vi "Write Message Queue.vi"(10 "Message Queue":refnum<class "JQMH_Message Queue.lvclass">, 11 "JQMHModule in":refnum<class "JQMHModule.lvclass">) -> (3 "JQMHModule out":refnum<class "JQMHModule.lvclass">)   [LabVIEW 2024, in "JQMHModule.lvclass"]
uses:
  JQMHModule.lvclass
  JQMHModule.lvclass/JQMHModule.ctl
  Message Queue_class/JQMH_Message Queue.lvclass
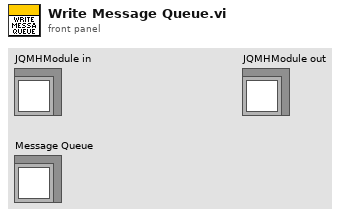
[diagram p1: front panel]
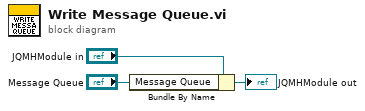
[diagram p0: block diagram]
diagram:
  n1 = Bundle By Name(cluster="JQMHModule in", "Message Queue"="Message Queue") -> (→"JQMHModule out":refnum<class "JQMHModule.lvclass">)
